vi "Increment Iteration Count.vi"(11 "Timing in":refnum<class "Engine Timing.lvclass">) -> (3 "Timing out":refnum<class "Engine Timing.lvclass">)   [LabVIEW 2017, in "Data Sharing Framework Core.lvlib" / "Data Sharing Framework Engine.lvlib" / "Engine Timing.lvclass"]
uses:
  Engine Timing.lvclass
  Engine Timing.lvclass/Engine Timing.ctl
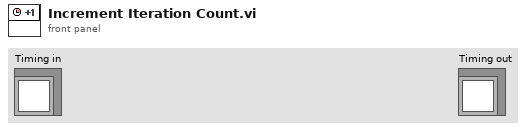
[diagram p1: front panel]
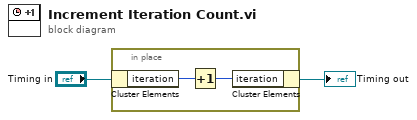
[diagram p0: block diagram]
diagram:
  n1 = in-place {
    n2 = in-place-cluster #1("Timing in") -> ("iteration"=w4:u64)
    n3 = Increment(x=w4) -> (x+1=w3:u64)
    n4 = in-place-cluster #1("iteration"=w3) -> (→"Timing out":refnum<class "Engine Timing.lvclass">)
  }
